vi "Write String.vi"(0 "NI Digital in":refnum<class "NI Analog Out.lvclass">, 1 "Bus In":refnum<class "Bus.lvclass">, 2 "Values":dbl[](array[numeric]), 3 "error in (no error)":errorcluster) -> (7 "NI Digital out":refnum<class "NI Analog Out.lvclass">, 8 "Bus Out":refnum<class "Bus.lvclass">, 10 "error out":errorcluster)   [LabVIEW 2018, in "NI Analog Out.lvclass"]
doc: "NI Analog Out.lvclass:Read String.vi\n\nThis is the Read String VI forthe NI Analog Out class.\n\nInstrument Communication Module Version 1.0\nOctober, 2020 Original Code Consulting Davita Bird\n www.originalcode.com"
uses:
  NI Analog Out.lvclass
  Bus/Bus.lvclass
  NI Analog Out.lvclass/NI Analog Out.ctl
  <vilib>/DAQmx/write.llb/DAQmx Write (Analog 1D DBL NChan 1Samp).vi
  <vilib>/DAQmx/miscellaneous.llb/DAQmx Fill In Error Info.vi
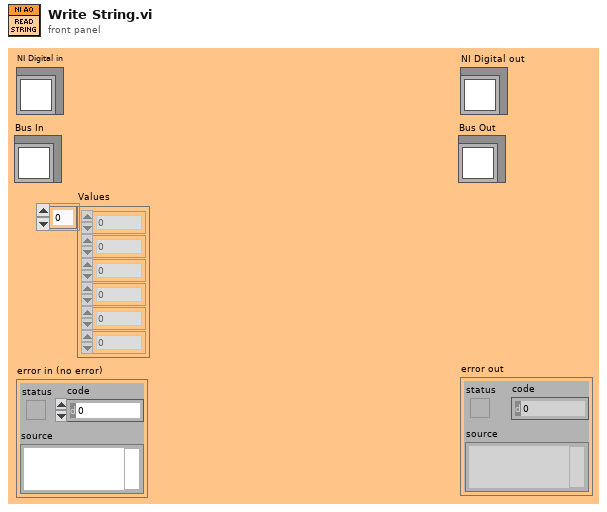
[diagram p1: front panel]
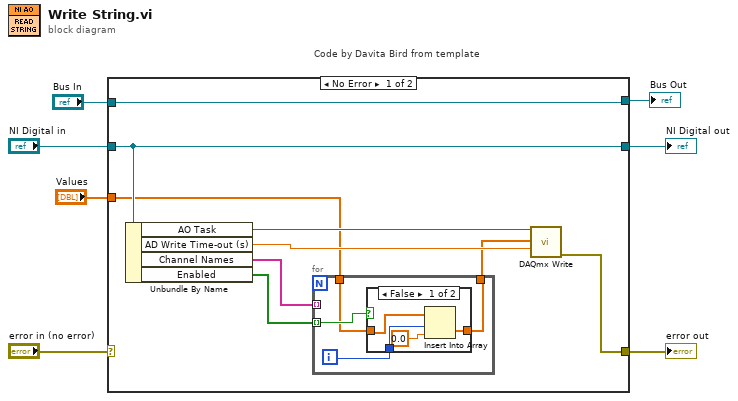
[diagram p0: block diagram]
diagram:
  n1 = case "Code by Davita Bird from template" shown="No Error" "error in (no error)" {
    selector: "error in (no error)" -> [_ w28]
    tunnel: [w13 w28] -> w6
    tunnel: [w15 w27] -> w5
    tunnel: "NI Digital in" -> [w15 w27]
    tunnel: "Values" -> [w9 _]
    tunnel: "Bus In" -> [w12 w26]
    tunnel: [w12 w26] -> w1
    frame No Error {
      n2 = Unbundle By Name(w15) -> ("AO Task"=w16:refnum<k21>, "AD Write Time-out (s)"=w14:dbl, "Channel Names"=w11:string[], "Enabled"=w10:bool[])
      n3 = for {
        tunnel: w11 -> [_] mode=indexing
        tunnel: w10 -> [w20] mode=indexing
        tunnel: w9 -> [w18]
        tunnel: [w19] -> w8
        i -> [w17]
        n4 = case shown="False" w20 {
          tunnel: [w24 w25] -> w19
          tunnel: w18 -> [w23 w25]
          tunnel: w17 -> [w22 _]
          frame False {
            n5 = Insert Into Array(array=w23, index=w22, new element=0.0 ("new element/subarray")) -> (w24:dbl[])
          }
          frame True {
          }
        }
      }
      n6 = call-poly <vilib>:"DAQmx Write.vi"("task/channels in"=w16, "data"=w8, "timeout"=w14) -> ("error out"=w13:errorcluster)  [unwired: 10 in, 2 out]
    }
    frame Error {
    }
  }
  "error out" <- w6
  "NI Digital out" <- w5
  "Bus Out" <- w1
